vi "OFBS_ArrayShuffle.vi"(1 "Array in":cluster{"ClassLabel":string, "Trial":dbl[][]}[](array[cluster])) -> (0 "Array out":cluster{"ClassLabel":string, "Trial":dbl[][]}[](array[cluster]))   [LabVIEW 2016, in "Optimal Frequency Bands Search.lvlib"]
doc: "Перетасовать элементы массива в случайном порядке"
uses:
  <vilib>/gmath/statdist.llb/Uniform (Discrete) Random.vi
  Optimal Frequency Bands Search.lvlib
  <vilib>/gmath/NI_Gmath.lvlib
panel:
  # "This VI is a part of BCI Design library, http://www.ru-bci.org \nCopyright © 2020, Sotnikov Peter, All rights reserved. License: CC BY-NC 4.0"
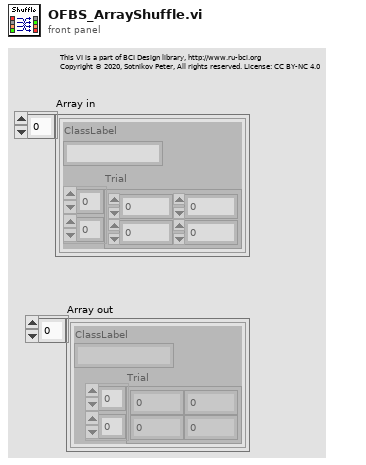
[diagram p1: front panel]
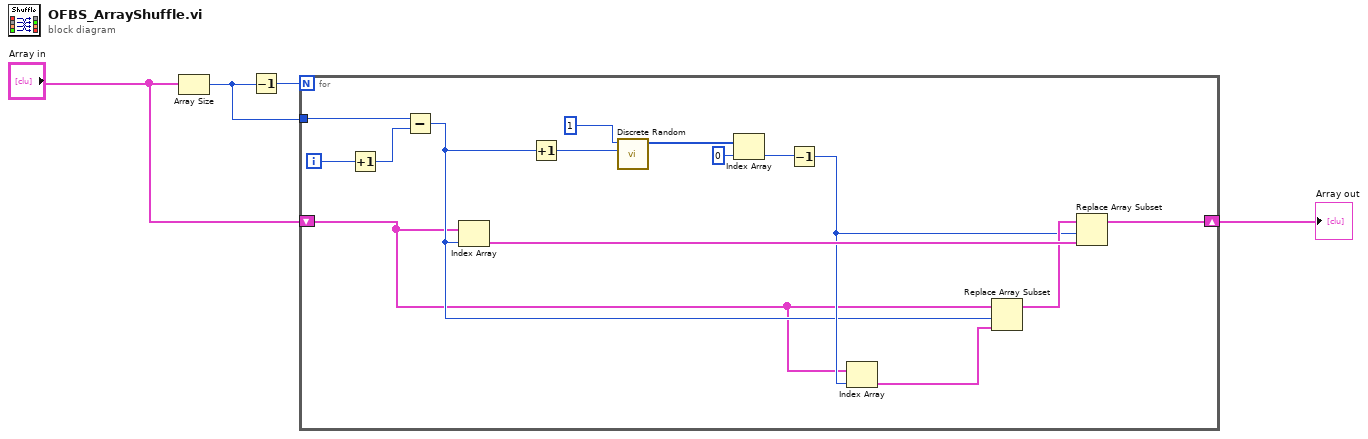
[diagram p0: block diagram]
diagram:
  n1 = Array Size(array="Array in") -> (size(s)=w3:i32)
  n2 = Decrement(x=w3) -> (x-1=w4:i32)
  n3 = for {
    N: w4 -> [_]
    tunnel: w3 -> [w7]
    shift-right: [w5] -> w1
    shift-left: "Array in" -> [w6]
    i -> [w19]
    n4 = Increment(x=w19) -> (x+1=w18:i32)
    n5 = Subtract(x=w7, y=w18) -> (x-y=w8:i32)
    n6 = Index Array "Index Array"(array=w6, index=w8) -> (element=w17:cluster{"ClassLabel":string, "Trial":dbl[][]})
    n7 = Increment(x=w8) -> (x+1=w11:i32)
    n8 = call-poly <vilib>:"Discrete Random.vi"("n"=w11, "samples"=1) -> ("uniform (discrete) random data"=w15:i32[])  [unwired: 8 in, 1 out]
    n9 = Index Array "Index Array"(array=w15, index=0) -> (element=w10:i32)
    n10 = Decrement(x=w10) -> (x-1=w9:i32)
    n11 = Index Array "Index Array"(array=w6, index=w9) -> (element=w13:cluster{"ClassLabel":string, "Trial":dbl[][]})
    n12 = Replace Array Subset "Replace Array Subset"(array=w6, new element=w13, index=w8) -> (w12:cluster{"ClassLabel":string, "Trial":dbl[][]}[])
    n13 = Replace Array Subset "Replace Array Subset"(array=w12, new element=w17, index=w9) -> (w5:cluster{"ClassLabel":string, "Trial":dbl[][]}[])
  }
  "Array out" <- w1
